vi "Test Cluster Data.vi"() -> ()   [LabVIEW 2021]
uses:
  Typedef/Cluster Info.ctl
  <vilib>/Utility/Data Type/Type Definitions/Data Type.ctl
  Typedef/Contiguous Structure for JSON Parse.ctl
  Typedef/Contiguous Structure.ctl
  Typedef/Endian.ctl
  Typedef/Element.ctl
  Typedef/Generic Datatypes.ctl
  DataTypes_CIF_U.lvlib
  <vilib>/Utility/Data Type/NI_Data Type.lvlib
panel:
  out "Pass":bool
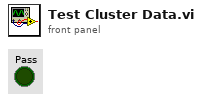
[diagram p1: front panel]
types:
  T1 = typedef "DataTypes_CIF_U.lvlib/Contiguous Structure.ctl" = cluster{"Endian":T2, "Array":bool, "Array Size":u32, "Element Size":u32, "struct_elems":T3[]}
  T2 = typedef "DataTypes_CIF_U.lvlib/Endian.ctl" = enum16{"Little Endian", "Big Endian"}
  T3 = typedef "Element.ctl" = cluster{"name":string, "type":T4, "size":u32, "offset":u32}
  T4 = typedef "DataTypes_CIF_U.lvlib/Generic Datatypes.ctl" = enum16{"Invalid", "Bool", "U8", "I8", "U16", "I16", "U32", "I32", "U64", "I64", "Single Float", "Double Float", "String"}
  T5 = typedef "DataTypes_CIF_U.lvlib/Contiguous Structure for JSON Parse.ctl" = cluster{"endianness":string, "array":bool, "arraysize":u32, "elemsize":u32, "struct_elems":cluster{"name":string, "type":string, "size":u32, "offset":u32}[]}
  T6 = cluster{"My number":i32, "next number":i32, "struct":cluster{"My number":i32, "Another":i32}, "Bool":bool}
  T7 = typedef "DataTypes_CIF_U.lvlib/Cluster Info.ctl" = cluster{"Name":string[], "Indices":i32[], "Type":T8, "Flat Data Size":u32, "Flat Data Offset":u32, "Memory Size":u32, "Memory Padding":u32, "Memory Offset":u32, "Type Descriptor":i16[]}
  T8 = typedef "NI_Data Type.lvlib/Data Type.ctl" = enum8{"Invalid Type", "Void", "I8", "I16", "I32", "I64", "U8", "U16", "U32", "U64", "Single Float", "Double Float", "Extended Float", "Single Complex", "Double Complex", "Extended Complex", "Enum U8", "Enum U16", "Enum U32", "Enum U64", "Single Float With Unit", "Double Float With Unit", "Extended Float With Unit", "Single Complex with Unit", "Double Complex with Unit", "Extended Complex with Unit", "Boolean", "String", "Path", "Picture", "Tag", "Array", "Cluster", "Variant", "LV Variant", "Waveform", "Timestamp", "Digital Waveform", "Digital Data", "ExpressData", "Refnum", "External Data", "VI", "Poly VI", "LabVIEW Class Instance", "Fixed Point", "Set Collection", "Map Collection"}
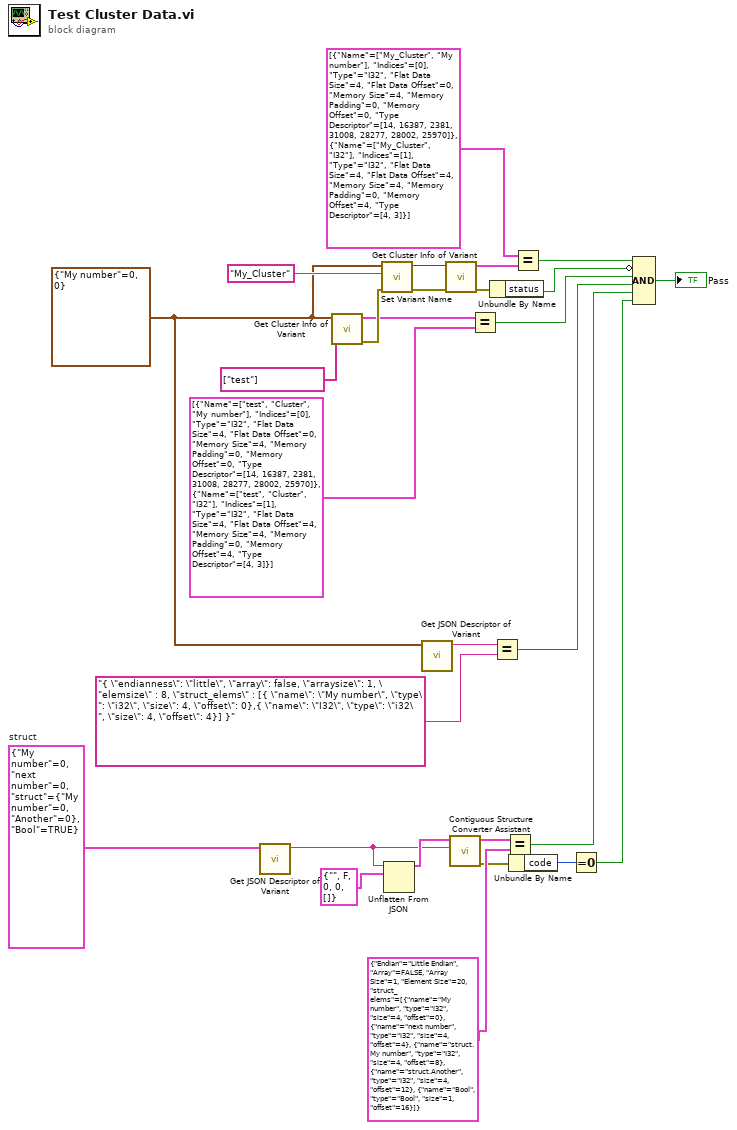
[diagram p0: block diagram]
diagram:
  w10 = T6 {"My number"=0, "next number"=0, "struct"={"My number"=0, "Another"=0}, "Bool"=TRUE}  # struct
  w14 = cluster{"My number":i32, i32} {"My number"=0, 0}
  n1 = call "Get JSON Descriptor of Variant.vi"("Data Type"=w10) -> ("JSON Descriptor"=w7:string)  [unwired: 8 in, 2 out]
  n2 = call "Get Cluster Info of Variant.vi"("Parent Name"=string[] ["test"], "Cluster Variant"=w14) -> ("error out"=w25:errorcluster, "Cluster Info"=w22:T7[])  [unwired: 5 in, 3 out]
  n3 = call "Set Variant Name.vi"("error in"=w25, "Name"="My_Cluster", "Variant_in"=w14) -> ("error out"=w24:errorcluster, "Variant_out"=w26:variant)  [unwired: 7 in]
  n4 = Unflatten From JSON(JSON string=w7, type and defaults=T5 {"endianness"="", "array"=FALSE, "arraysize"=0, "elemsize"=0, "struct_elems"=[]} ("Contiguous Structure from JSON Parse")) -> (value=w8:T5)  [unwired: 5 in, 1 out]
  n5 = call "Get JSON Descriptor of Variant.vi"("Data Type"=w14) -> ("JSON Descriptor"=w13:string)  [unwired: 8 in, 2 out]
  n6 = call "Get Cluster Info of Variant.vi"("error in (no error)"=w24, "Cluster Variant"=w26) -> ("error out"=w18:errorcluster, "Cluster Info"=w20:T7[])  [unwired: 5 in, 3 out]
  n7 = call "Contiguous Structure Converter Assistant.vi"("Original JSON"=w7, "Contiguous Structure from JSON Parse"=w8) -> ("error out"=w3:errorcluster, "Contiguous Structure"=w6:T1)  [unwired: 8 in]
  n8 = Equal?(x=w22, y=T7[] [{"Name"=["test", "Cluster", "My number"], "Indices"=[0], "Type"=enum."I32", "Flat Data Size"=4, "Flat Data Offset"=0, "Memory Size"=4, "Memory Padding"=0, "Memory Offset"=0, "Type Descriptor"=[14, 16387, 2381, 31008, 28277, 28002, 25970]}, {"Name"=["test", "Cluster", "I32"], "Indices"=[1], "Type"=enum."I32", "Flat Data Size"=4, "Flat Data Offset"=4, "Memory Size"=4, "Memory Padding"=0, "Memory Offset"=4, "Type Descriptor"=[4, 3]}] ("Cluster Info 3")) -> (x = y?=w15:bool)
  n9 = Unbundle By Name(w18) -> ("status"=w16:bool)
  n10 = Equal?(x=w13, y="{ \"endianness\": \"little\", \"array\": false, \"arraysize\": 1, \"elemsize\" : 8, \"struct_elems\" : [{ \"name\": \"My number\", \"type\": \"i32\", \"size\": 4, \"offset\": 0},{ \"name\": \"I32\", \"type\": \"i32\", \"size\": 4, \"offset\": 4}] }" ("JSON Descriptor 2")) -> (x = y?=w11:bool)
  n11 = Equal?(x=w6, y=T1 {"Endian"=enum."Little Endian", "Array"=FALSE, "Array Size"=1, "Element Size"=20, "struct_elems"=[{"name"="My number", "type"=enum."I32", "size"=4, "offset"=0}, {"name"="next number", "type"=enum."I32", "size"=4, "offset"=4}, {"name"="struct.My number", "type"=enum."I32", "size"=4, "offset"=8}, {"name"="struct.Another", "type"=enum."I32", "size"=4, "offset"=12}, {"name"="Bool", "type"=enum."Bool", "size"=1, "offset"=16}]} ("Contiguous Structure")) -> (x = y?=w4:bool)
  n12 = Unbundle By Name(w3) -> ("code"=w2:i32)
  n13 = Equal?(x=T7[] [{"Name"=["My_Cluster", "My number"], "Indices"=[0], "Type"=enum."I32", "Flat Data Size"=4, "Flat Data Offset"=0, "Memory Size"=4, "Memory Padding"=0, "Memory Offset"=0, "Type Descriptor"=[14, 16387, 2381, 31008, 28277, 28002, 25970]}, {"Name"=["My_Cluster", "I32"], "Indices"=[1], "Type"=enum."I32", "Flat Data Size"=4, "Flat Data Offset"=4, "Memory Size"=4, "Memory Padding"=0, "Memory Offset"=4, "Type Descriptor"=[4, 3]}] ("Cluster Info"), y=w20) -> (x = y?=w17:bool)
  n14 = Equal To 0?(x=w2) -> (x = 0?=w1:bool)
  n15 = Compound Arithmetic op=AND(w17, invert w16, w15, w11, w4, w1) -> (→"Pass":bool)
